vi "execute.vi"(8 "error in (no error)":errorcluster, 9 "ParameterString":string, 10 "ObjectCluster":T1, 11 "OutDoorLightCommand in":refnum<class "OutDoorLightCommand.lvclass">) -> (0 "error out":errorcluster, 2 "ObjectCluster Out":T1, 3 "OutDoorLightCommand out":refnum<class "OutDoorLightCommand.lvclass">)   [LabVIEW 2013, in "OutDoorLightCommand.lvclass"]
uses:
  OutDoorLightCommand.lvclass
  Command.lvclass/ObjectCluster.ctl
  AirCondition.lvclass/AirCondition.lvclass
  RoomLight.lvclass/RoomLight.lvclass
  OutDoorLight.lvclass/OutDoorLight.lvclass
  Television.lvclass/Television.lvclass
  Stereo.lvclass/Stereo.lvclass
  Command.lvclass/Command.lvclass
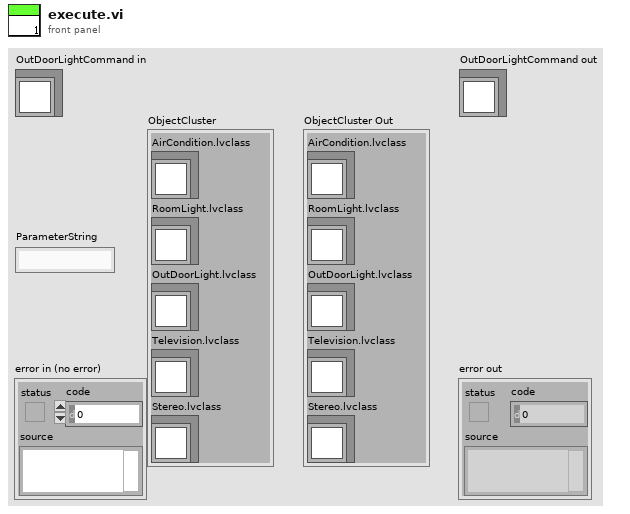
[diagram p1: front panel]
types:
  T1 = typedef "Command.lvclass/ObjectCluster.ctl" = cluster{"AirCondition.lvclass":refnum<class "AirCondition.lvclass">, "RoomLight.lvclass":refnum<class "RoomLight.lvclass">, "OutDoorLight.lvclass":refnum<class "OutDoorLight.lvclass">, "Television.lvclass":refnum<class "Television.lvclass">, "Stereo.lvclass":refnum<class "Stereo.lvclass">}
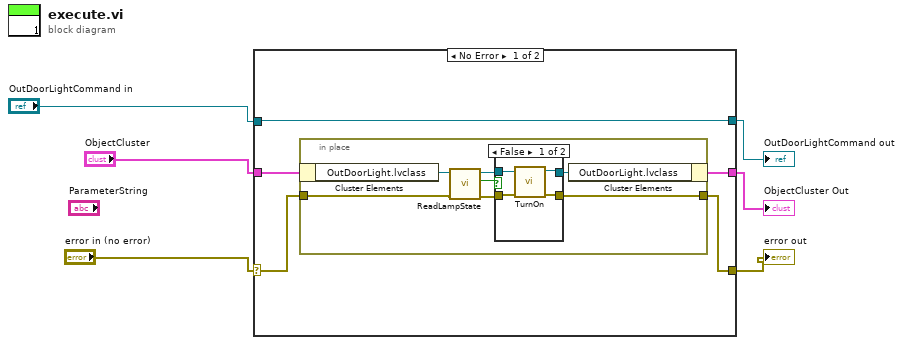
[diagram p0: block diagram]
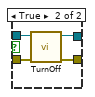
[diagram p2: hidden frame]
diagram:
  n1 = case shown="No Error" "error in (no error)" {
    selector: "error in (no error)" -> [w10 w27]
    tunnel: "ObjectCluster" -> [w11 w28]
    tunnel: "OutDoorLightCommand in" -> [w7 w29]
    tunnel: [w9 w27] -> w4
    tunnel: [w8 w28] -> w5
    tunnel: [w7 w29] -> w6
    frame No Error {
      n2 = in-place {
        in-place-border: w10 -> [w15]
        in-place-border: [w17] -> w9
        n3 = in-place-cluster #1(w11) -> ("OutDoorLight.lvclass"=w16:refnum<class "OutDoorLight.lvclass">)
        n4 = call-dynamic "ReadLampState.vi"("error in (no error)"=w15, "OutDoorLight in"=w16) -> ("error out"=w14:errorcluster, "LampState"=w12:bool, "OutDoorLight out"=w13:refnum<class "OutDoorLight.lvclass">)  [unwired: 7 in]
        n5 = case shown="False" w12 {
          tunnel: w13 -> [w21 w25]
          tunnel: w14 -> [w22 w26]
          tunnel: [w20 w24] -> w18
          tunnel: [w19 w23] -> w17
          frame False {
            n6 = call-dynamic "TurnOn.vi"("error in (no error)"=w22, "OutDoorLight in"=w21) -> ("error out"=w19:errorcluster, "OutDoorLight out"=w20:refnum<class "OutDoorLight.lvclass">)  [unwired: 8 in]
          }
          frame True {
            n7 = call-dynamic "TurnOff.vi"("error in (no error)"=w26, "OutDoorLight in"=w25) -> ("error out"=w23:errorcluster, "OutDoorLight out"=w24:refnum<class "OutDoorLight.lvclass">)  [unwired: 8 in]
          }
        }
        n8 = in-place-cluster #1("OutDoorLight.lvclass"=w18) -> (w8:T1)
      }
    }
    frame Error {
    }
  }
  "error out" <- w4
  "OutDoorLightCommand out" <- w6
  "ObjectCluster Out" <- w5
